vi "FITS hdr gen row str.vi"(5 "Format":string, 9 "Comment":string, 10 "Value":string, 11 "Field":string) -> (3 "FITS Row":string)   [LabVIEW 2022 SP3]
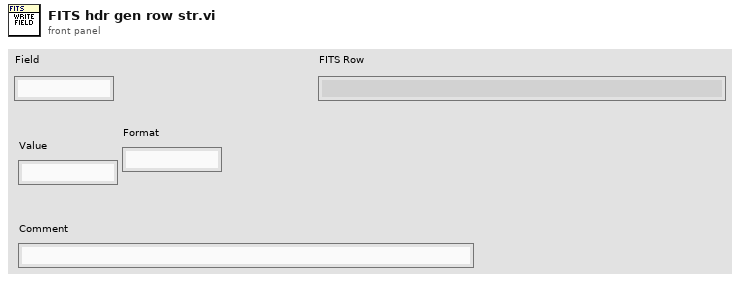
[diagram p1: front panel]
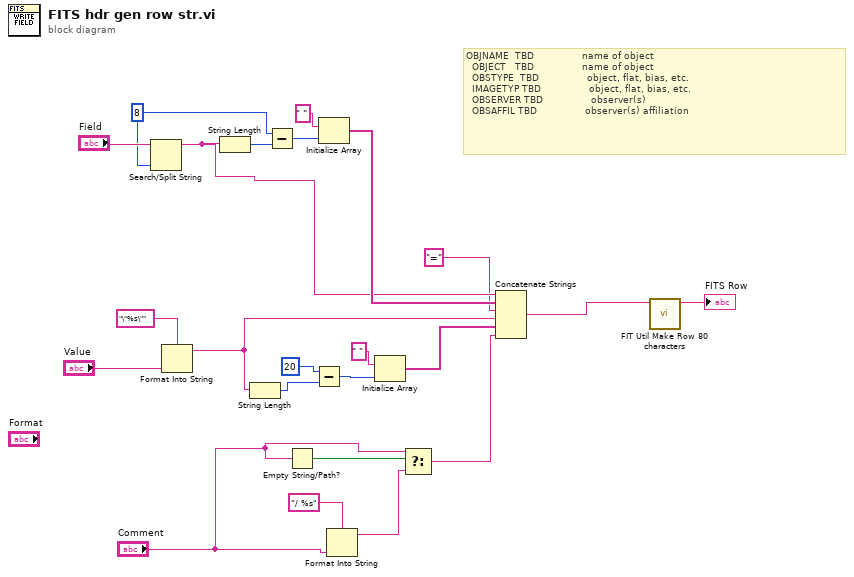
[diagram p0: block diagram]
diagram:
  w22 = 8
  # "OBJNAME  TBD                name of object\n  OBJECT   TBD                name of object\n  OBSTYPE  TBD                object, flat, bias, etc.\n  IMAGETYP TBD                object, flat, bias, etc.\n  OBSERVER TBD                observer(s) \n  OBSAFFIL TBD                observer(s) affiliation"
  n1 = Search/Split String(string="Field", offset (0)=w22) -> (substring before match=w2:string)  [unwired: 1 in, 2 out]
  n2 = Format Into String(format string="\"%s\"", "Value") -> (resulting string=w9:string)  [unwired: 2 in, 1 out]
  n3 = String Length(string=w2) -> (length=w21:i32)
  n4 = String Length(string=w9) -> (length=w11:i32)
  n5 = Subtract(x=w22, y=w21) -> (x-y=w20:i32)
  n6 = Empty String/Path?(string/path="Comment") -> (empty?=w6:bool)
  n7 = Subtract(x=20, y=w11) -> (x-y=w8:i32)
  n8 = Initialize Array(" ", w20) -> (w17:string[])
  n9 = Format Into String(format string="/ %s", "Comment") -> (resulting string=w4:string)  [unwired: 2 in, 1 out]
  n10 = Initialize Array(" ", w8) -> (w7:string[])
  n11 = Select(t="Comment", s=w6, f=w4) -> (s? t:f=w3:string)
  n12 = Concatenate Strings(w2, w17, "=" ("string"), w9, w7, w3) -> (w10:string)
  n13 = call "FIT Util Make Row 80 characters.vi"("Row"=w10) -> ("Row with 80 char"=→"FITS Row":string)  [unwired: 10 in]
